vi "22 RESTful API.vi"() -> ()   [LabVIEW 2024]
uses:
  <userlib>/1. Examples/_Subs/OpenDiagram/Open_XControl.xctl
  <vilib>/httpClient/LabVIEWHTTPClient.lvlib
panel:
  out "Property (str)":string
  in  "OpenDiag":refnum<vi>(xcontrol)
  # "02 RESTful API\nThis code goes online to get a Chuck Norris Joke \n\nInstructions:\n1. Connect your computer to the internet\n2. Hit Run and read the joke"
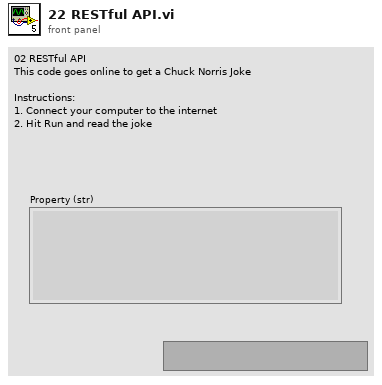
[diagram p1: front panel]
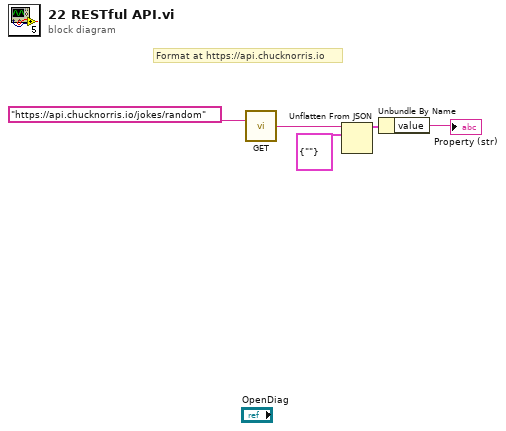
[diagram p0: block diagram]
diagram:
  # "Format at https://api.chucknorris.io"
  n1 = call <vilib>:"GET.vi"("url"="https://api.chucknorris.io/jokes/random") -> ("body"=w4:string)  [unwired: 11 in, 3 out]
  n2 = Unflatten From JSON(JSON string=w4, type and defaults=cluster{"value":string} {"value"=""}) -> (value=w2:cluster{"value":string})  [unwired: 5 in, 1 out]
  n3 = Unbundle By Name(w2) -> ("value"=→"Property (str)":string)
